vi "LabViewTest.vi"() -> ()   [LabVIEW 2022 SP3]
uses:
  build/liblib.so
panel:
  out "return type 2":string
  out "error out":errorcluster
  in  "return type":string
  in  "error in (no error)":errorcluster
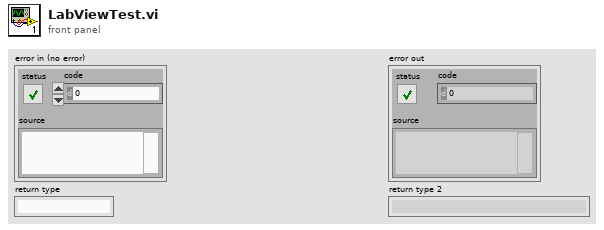
[diagram p1: front panel]
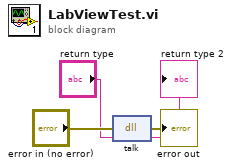
[diagram p0: block diagram]
diagram:
  n1 = dll-call lib="home/vlad/Desktop/opendaq/opendaq-3.0.0-examples/cpp/Dynamic Lib example/build/liblib.so" fn="talk"(error in="error in (no error)", "return type"="return type") -> (error out=→"error out":errorcluster, "return type"=→"return type 2":string)  [unwired: 1 in, 1 out]
